vi "BRig_dataCurrent_T_Cue2_LED_start.vi"() -> (2 "output_T_Cue2_LED_start":i32)   [LabVIEW 2014]
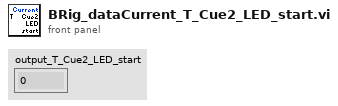
[diagram p1: front panel]
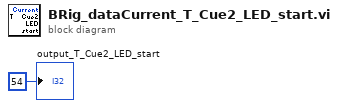
[diagram p0: block diagram]
diagram:
  "output_T_Cue2_LED_start" <- 54 ("output_iBlock")
